vi "hydrolyse_reactor_parallel.vi"(2 "Instances":i16, 4 "Dataflow In":errorcluster) -> (1 "Dataflow Out":errorcluster)   [LabVIEW 2019]
uses:
  lib/libSimulationControl/libSimulationControl.lvlib
panel:
  # "*******************************************************************\nBiogas Plant Control\n\nAuthor: Paul Zügel\nGCSC-Frankfurt am Main 2020\n\n*******************************************************************"
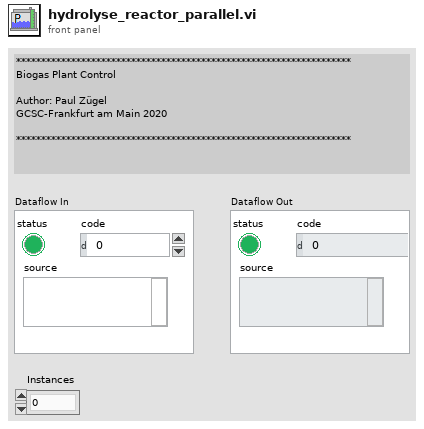
[diagram p1: front panel]
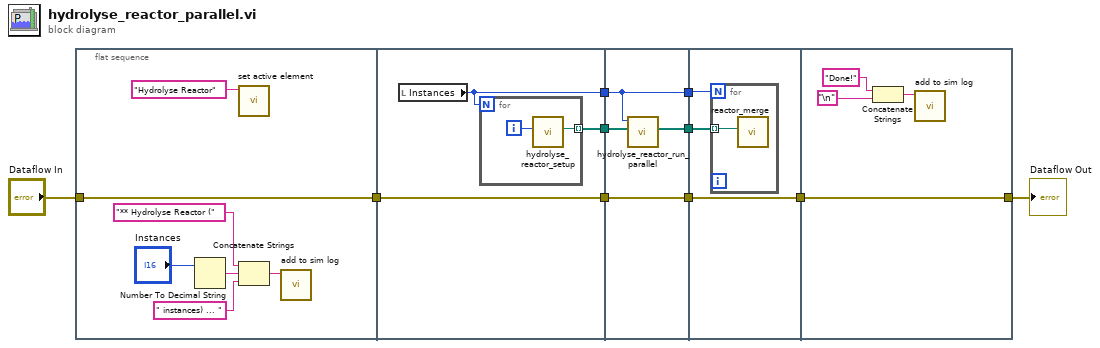
[diagram p0: block diagram]
diagram:
  n1 = flat-sequence {
    tunnel: [w17] -> w9
    tunnel: "Dataflow In" -> [w17]
    tunnel: [w20] -> w6
    tunnel: w9 -> [w20]
    tunnel: [w19] -> w4
    tunnel: [w18] -> w3
    tunnel: w6 -> [w26]
    tunnel: [w26] -> w5
    tunnel: w4 -> [w23]
    tunnel: w3 -> [w25]
    tunnel: [w24] -> w2
    tunnel: [w23] -> w1
    tunnel: w5 -> [w29]
    tunnel: [w29] -> w7
    tunnel: w2 -> [w28]
    tunnel: w1 -> [w27]
    tunnel: [w34] -> w8
    tunnel: w7 -> [w34]
    frame #0 {
      n2 = Number To Decimal String(number="Instances") -> (decimal integer string=w15:string)  [unwired: 1 in]
      n3 = call "set active element.vi"("elem"="Hydrolyse Reactor") -> ()  [unwired: 10 in, 1 out]
      n4 = Concatenate Strings("** Hydrolyse Reactor (" ("string"), w15, " instances) ... " ("string")) -> (w13:string)
      n5 = call "add to sim log.vi"("log"=w13) -> ()  [unwired: 10 in, 1 out]
    }
    frame #1 {
      n6 = local read "Instances"() -> (w19:i16)
      n7 = for {
        N: w19 -> [_]
        tunnel: [w21] -> w18 mode=indexing
        i -> [w22]
        n8 = call "hydrolyse_reactor_setup.vi"("#"=w22) -> ("spec_file"=w21:path)  [unwired: 10 in]
      }
    }
    frame #2 {
      n9 = call "hydrolyse_reactor_run_parallel.vi"("Spec files"=w25, "instances"=w23) -> ("paths out"=w24:path[])  [unwired: 9 in]
    }
    frame #3 {
      n10 = for {
        N: w27 -> [_]
        tunnel: w28 -> [w30] mode=indexing
        n11 = call "reactor_merge.vi"("reactor_path"=w30) -> ()  [unwired: 11 in]
      }
    }
    frame #4 {
      n12 = Concatenate Strings("Done!" ("string"), "\n") -> (w31:string)
      n13 = call "add to sim log.vi"("log"=w31) -> ()  [unwired: 10 in, 1 out]
    }
  }
  "Dataflow Out" <- w8
